vi "_write.vi"(1 "数据输入":string, 2 "连接ID":refnum<k5>) -> (0 "连接ID输出":refnum<k5>)   [LabVIEW 2017]
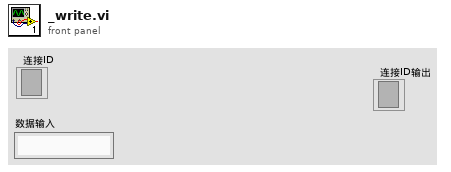
[diagram p1: front panel]
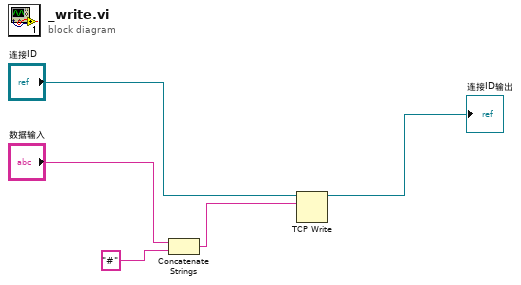
[diagram p0: block diagram]
diagram:
  n1 = Concatenate Strings("数据输入", "#" ("字符串")) -> (w4:string)
  n2 = TCP Write(connection ID="连接ID", data in=w4) -> (connection ID out=→"连接ID输出":refnum<k5>)  [unwired: 2 in, 2 out]
